vi "Convert Byte Array to U32 RGBA Array.vi"(8 "error in (no error)":errorcluster, 10 "FrameDescription":T1, 11 "Byte Array":u8[](array[numeric])) -> (0 "error out":errorcluster, 3 "RGBA U32 Array":u32[][](array[numeric]))   [LabVIEW 2014]
uses:
  controls/FrameDescription.ctl
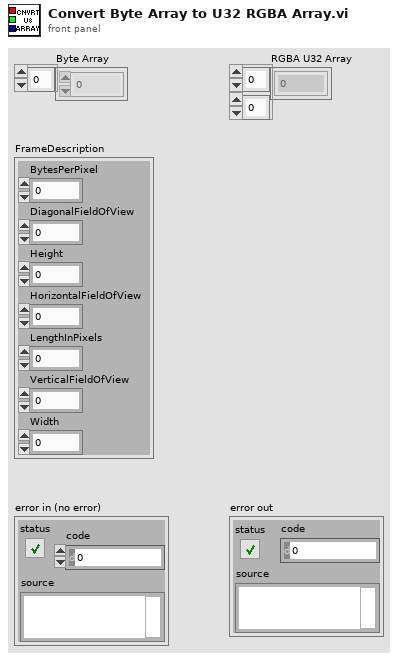
[diagram p1: front panel]
types:
  T1 = typedef "FrameDescription.ctl" = cluster{"BytesPerPixel":u32, "DiagonalFieldOfView":sgl, "Height":i32, "HorizontalFieldOfView":sgl, "LengthInPixels":u32, "VerticalFieldOfView":sgl, "Width":i32}
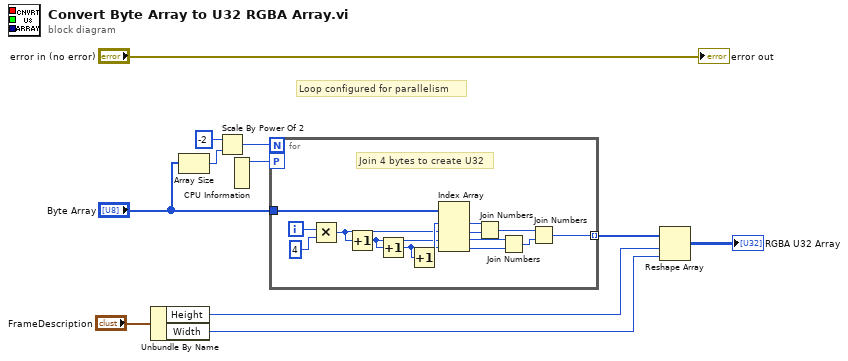
[diagram p0: block diagram]
diagram:
  # "Loop configured for parallelism"
  n1 = Unbundle By Name("FrameDescription") -> ("Height"=w3:i32, "Width"=w2:i32)
  n2 = Array Size(array="Byte Array") -> (size(s)=w8:i32)
  n3 = Scale By Power Of 2(n=i16 -2, x=w8) -> (x*2^n=w9:i32)
  n4 = CPU Information() -> (4:w4:i32)  [unwired: 3 out]
  n5 = for {
    N: w9 -> [_]
    tunnel: "Byte Array" -> [w25]
    tunnel: [w16] -> w10 mode=indexing
    workers-P: w4 -> [_]
    i -> [w24]
    # "Join 4 bytes to create U32"
    n6 = Multiply(x=w24, y=4) -> (x*y=w14:i32)
    n7 = Increment(x=w14) -> (x+1=w13:i32)
    n8 = Increment(x=w13) -> (x+1=w12:i32)
    n9 = Increment(x=w12) -> (x+1=w15:i32)
    n10 = Index Array(array=w25, index #1=w15, index #2=w14, index #3=w13, index #4=w12) -> (element #1=w22:u8, element #2=w21:u8, element #3=w20:u8, element #4=w17:u8)
    n11 = Join Numbers(hi=w22, lo=w21) -> ((hi.lo)=w19:u16)
    n12 = Join Numbers(hi=w20, lo=w17) -> ((hi.lo)=w18:u16)
    n13 = Join Numbers(hi=w19, lo=w18) -> ((hi.lo)=w16:u32)
  }
  n14 = Reshape Array(w10, w3, w2) -> (→"RGBA U32 Array":u32[][])
  "error out" <- "error in (no error)"
